vi "Load Settings.vi"(4 "Controls[]":refnum<vi>[](array[refnum]), 7 "VI Refnum":refnum<vi>, 8 "error in (no error)":errorcluster, 9 "Section":string, 10 "Path":path, 11 "Save Restore Settings in":refnum<class "Save Restore Settings.lvclass">) -> (0 "error out":errorcluster, 3 "Save Restore Settings out":refnum<class "Save Restore Settings.lvclass">)   [LabVIEW 2016, in "Save Restore Settings.lvclass"]
uses:
  <userlib>/_MGI/Application Control/MGI Save Restore Settings/Save Restore Settings.lvclass
  <userlib>/_MGI/Application Control/MGI Save Restore Settings/Save Restore Settings.lvclass/Save Restore Settings.ctl
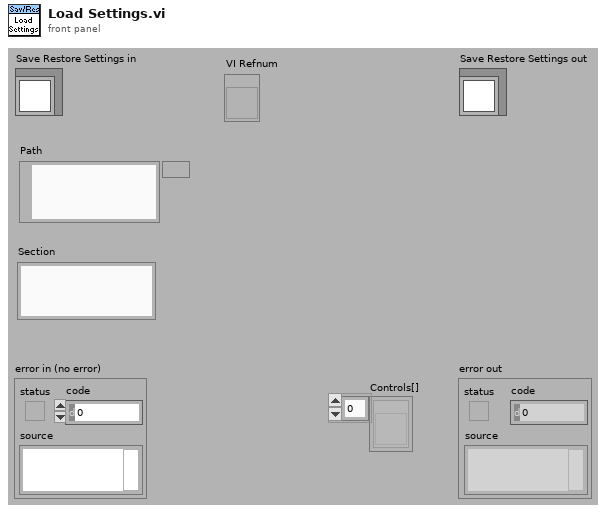
[diagram p1: front panel]
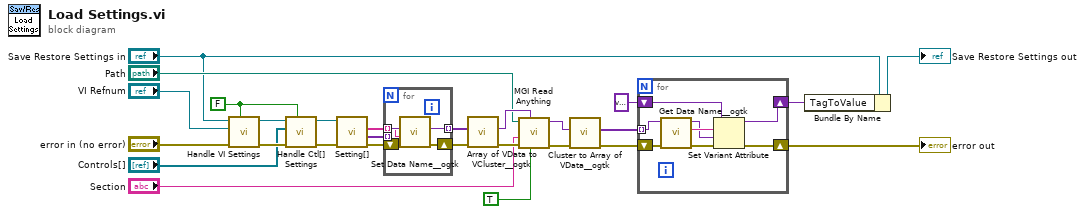
[diagram p0: block diagram]
diagram:
  w2 = FALSE ("Write VI? (F:Read)")
  n1 = call-dynamic "Handle VI Settings.vi"("Write VI? (F:Read)"=w2, "error in (no error)"="error in (no error)", "VI Refnum"="VI Refnum", "Save Restore Settings in"="Save Restore Settings in") -> ("error out"=w19:errorcluster, "Save Restore Settings out"=w22:refnum<class "Save Restore Settings.lvclass">)  [unwired: 6 in]
  n2 = call-dynamic "Handle Ctl[] Settings.vi"("Write Ctl? (F:Read)"=w2, "error in (no error)"=w19, "Controls[]"="Controls[]", "Save Restore Settings in"=w22) -> ("error out"=w18:errorcluster, "Save Restore Settings out"=w17:refnum<class "Save Restore Settings.lvclass">)  [unwired: 6 in]
  n3 = call-dynamic "Setting[].vi"("error in (no error)"=w18, "Save Restore Settings in"=w17) -> ("error out"=w27:errorcluster, "Value[]"=w26:variant[], "Tag[]"=w25:string[])  [unwired: 6 in, 1 out]
  n4 = for {
    shift-right: [w29] -> w23
    shift-left: w27 -> [w32]
    tunnel: w26 -> [w31] mode=indexing
    tunnel: w25 -> [w30] mode=indexing
    tunnel: [w28] -> w24 mode=indexing
    n5 = call <userlib>:"Set Data Name__ogtk.vi"("error in (no error)"=w32, "Data Name"=w30, "Data"=w31) -> ("error out"=w29:errorcluster, "Renamed Data"=w28:variant)  [unwired: 7 in]
  }
  n6 = call <userlib>:"Array of VData to VCluster__ogtk.vi"("error in (no error)"=w23, "Array"=w24) -> ("error out"=w16:errorcluster, "VCluster"=w15:variant)  [unwired: 8 in]
  n7 = call <userlib>:"MGI Read Anything.vi"("Use Supplied (F: Use Default)"=TRUE, "Type of Anything"=w15, "Error In"=w16, "Section Name (Name of \"Type of Anything\")"="Section", "Path (dialog)"="Path") -> ("Error Out"=w14:errorcluster, "Anything"=w13:variant)  [unwired: 3 in, 2 out]
  n8 = call <userlib>:"Cluster to Array of VData__ogtk.vi"("error in (no error)"=w14, "Cluster"=w13) -> ("error out"=w12:errorcluster, "Array of VData"=w11:variant[])  [unwired: 8 in]
  n9 = for {
    shift-right: [w37] -> w4
    shift-left: w12 -> [w39]
    tunnel: w11 -> [w40] mode=indexing
    shift-right: [w34] -> w6
    shift-left: variant -> [w33]
    n10 = call <userlib>:"Get Data Name__ogtk.vi"("error in (no error)"=w39, "Data"=w40) -> ("error out"=w38:errorcluster, "Data Name"=w36:string, "Data dup"=w35:variant)  [unwired: 7 in]
    n11 = Set Variant Attribute(Variant=w33, name=w36, value=w35, error in=w38) -> (Variant out=w34:variant, error out=w37:errorcluster)  [unwired: 1 out]
  }
  "error out" <- w4
  n12 = Bundle By Name(cluster="Save Restore Settings in", "TagToValue"=w6) -> (→"Save Restore Settings out":refnum<class "Save Restore Settings.lvclass">)
